vi "String To TimeStamp.vi"(6 "Type":enum16{"h:m:s", "Y-M-D h:m:s"}(ring), 8 "error in":errorcluster, 11 "Time string":string) -> (0 "error out":errorcluster, 3 "Time Stamp":timestamp)   [LabVIEW 2016]
uses:
  <vilib>/Utility/miscctls.llb/LVDateTimeRec.ctl
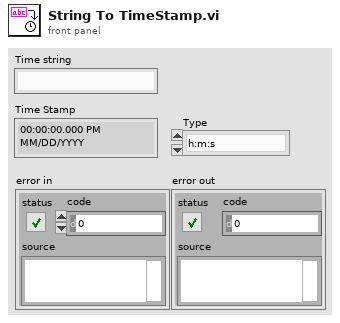
[diagram p1: front panel]
types:
  T1 = typedef "LVDateTimeRec.ctl" = cluster{"fractional second":dbl, "second":i32, "minute":i32, "hour":i32, "day of month":i32, "month":i32, "year":i32, "day of week":i32, "day of year":i32, "DST":i32}
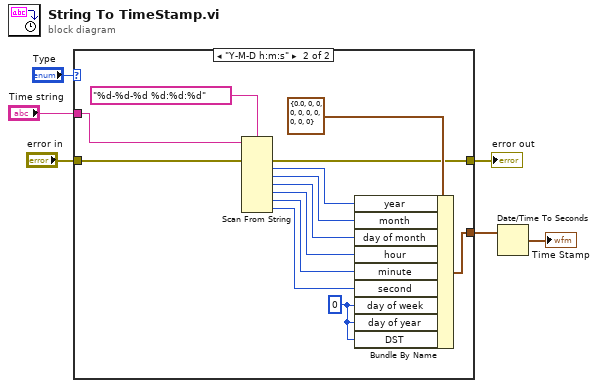
[diagram p0: block diagram]
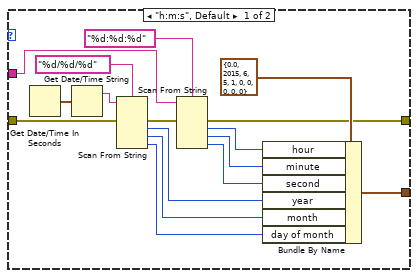
[diagram p2: hidden frame]
diagram:
  n1 = case shown="\"Y-M-D h:m:s\"" "Type" {
    tunnel: "Time string" -> [w22 w35]
    tunnel: [w17 w26] -> w4
    tunnel: "error in" -> [w11 w25]
    tunnel: [w16 w23] -> w1
    frame "h:m:s", Default {
      n2 = Get Date/Time In Seconds() -> (seconds since 1Jan1904=w12:timestamp)
      n3 = Get Date/Time String(seconds (now)=w12) -> (date string=w13:string)  [unwired: 2 in, 1 out]
      n4 = Scan From String(format string="%d/%d/%d", input string=w13, error in=w11) -> (error out=w10:errorcluster, output 1=w9:i32, output 2=w8:i32, output 3=w7:i32)  [unwired: 4 in, 2 out]
      n5 = Scan From String(format string="%d:%d:%d", input string=w22, error in=w10) -> (error out=w16:errorcluster, output 1=w20:i32, output 2=w19:i32, output 3=w18:i32)  [unwired: 4 in, 2 out]
      n6 = Bundle By Name(cluster=T1 {"fractional second"=0.0, "second"=2015, "minute"=6, "hour"=5, "day of month"=1, "month"=0, "year"=0, "day of week"=0, "day of year"=0, "DST"=0} ("date time rec"), "hour"=w20, "minute"=w19, "second"=w18, "year"=w9, "month"=w8, "day of month"=w7) -> (w17:T1)
    }
    frame "Y-M-D h:m:s" {
      w28 = 0
      n7 = Scan From String(format string="%d-%d-%d %d:%d:%d", input string=w35, error in=w25) -> (error out=w23:errorcluster, output 1=w34:i32, output 2=w33:i32, output 3=w32:i32, output 4=w31:i32, output 5=w30:i32, output 6=w29:i32)  [unwired: 7 in, 2 out]
      n8 = Bundle By Name(cluster=T1 {"fractional second"=0.0, "second"=0, "minute"=0, "hour"=0, "day of month"=0, "month"=0, "year"=0, "day of week"=0, "day of year"=0, "DST"=0} ("date time rec"), "year"=w34, "month"=w33, "day of month"=w32, "hour"=w31, "minute"=w30, "second"=w29, "day of week"=w28, "day of year"=w28, "DST"=w28) -> (w26:T1)
    }
  }
  "error out" <- w1
  n9 = Date/Time To Seconds(2:w4) -> (0:→"Time Stamp":timestamp)  [unwired: 1 in]
